vi "DEMO.vi"() -> ()   [LabVIEW 2013]
doc: "Use this template to build a producer/consumer design pattern with events to produce queue items. Use this design pattern instead of the User Interface Event Handler pattern for user interfaces when you want to execute code asynchronously in response to an event without slowing the user interface responsiveness."
uses:
  GumballMachine.lvclass/GumballMachine.lvclass
  ActionMark.ctl
panel:
  in  "Charge":bool
  out "ProcessMessage":string
  in  "TurnCrank":bool
  in  "EjectCoin":bool
  in  "InsertCoin":bool
  # "狀態模式簡例"
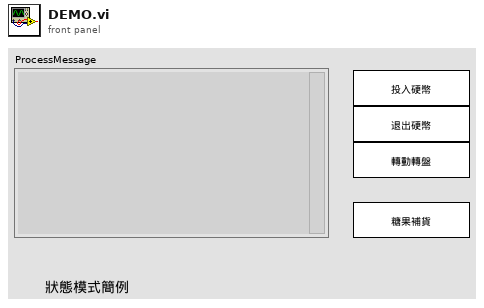
[diagram p1: front panel]
types:
  T1 = typedef "ActionMark.ctl" = enum16{"投入硬幣", "退回硬幣", "轉動轉盤", "糖果補貨"}
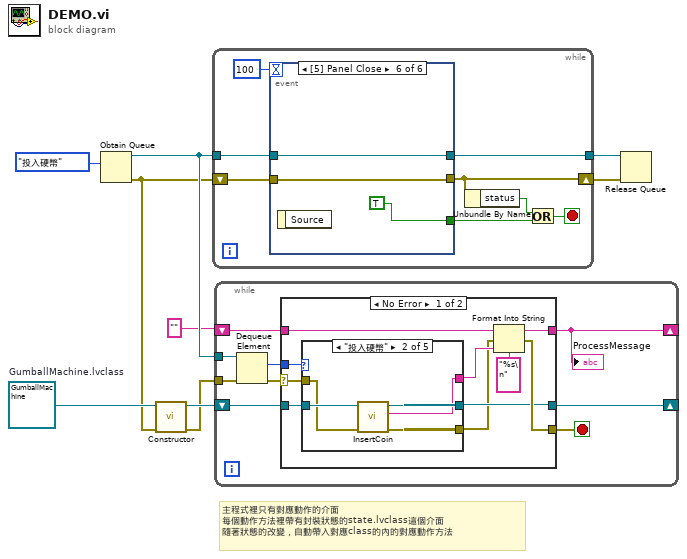
[diagram p0: block diagram]
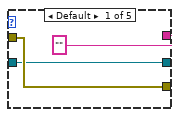
[diagram p2: hidden frame]
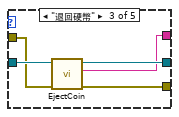
[diagram p3: hidden frame]
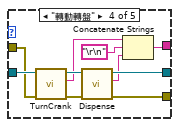
[diagram p4: hidden frame]
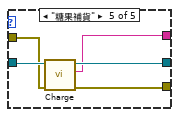
[diagram p5: hidden frame]
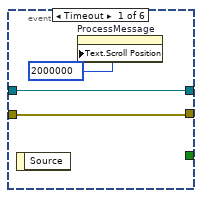
[diagram p7: hidden frame]
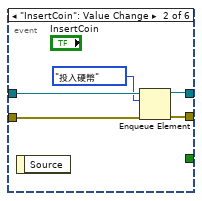
[diagram p8: hidden frame]
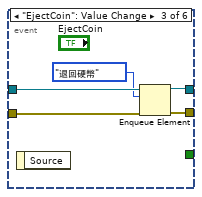
[diagram p9: hidden frame]
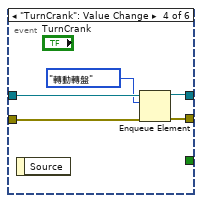
[diagram p10: hidden frame]
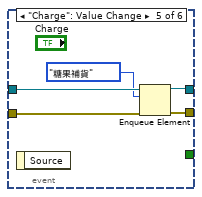
[diagram p11: hidden frame]
diagram:
  w5 = refnum<class "GumballMachine.lvclass"> refnum  # GumballMachine.lvclass
  # "主程式裡只有對應動作的介面\n每個動作方法裡帶有封裝狀態的state.lvclass這個介面\n隨著狀態的改變，自動帶入對應class的內的對應動作方法"
  n1 = Obtain Queue(element data type=ActionMark."投入硬幣" ("State")) -> (queue out=w8:refnum<queue>, error out=w2:errorcluster)  [unwired: 4 in, 1 out]
  n2 = call "Constructor.vi"("error in (no error)"=w2, "GumballMachine in"=w5) -> ("error out"=w3:errorcluster, "GumballMachine out"=w4:refnum<class "GumballMachine.lvclass">)  [unwired: 8 in]
  n3 = while {
    shift-right: [w13] -> w9
    shift-left: w2 -> [w16]
    tunnel: w8 -> [w17]
    tunnel: [w11] -> w6
    stop <- w14 stop-if-true
    n4 = event shown="[5] Panel Close" {
      selector: _ -> [_ _ _ _ _ _]
      dyn-events: _ -> [_ _ _ _ _ _]
      timeout: 100 -> [_ _ _ _ _ _]
      tunnel: w17 -> [w19 w25 w30 w35 w40 w41]
      tunnel: w16 -> [w20 w24 w29 w34 w39 w43]
      tunnel: [w20 w23 w28 w33 w38 w43] -> w13
      tunnel: [_ _ _ _ _ TRUE ("stop")] -> w15
      tunnel: [w19 w21 w26 w31 w36 w41] -> w11
      event Timeout {
        n5 = event-data() -> ()  [unwired: 1 in, 1 out]
        n6 = property on="ProcessMessage" class="Str"("Text.Scroll Position"=u32 2000000) -> ()  [unwired: 2 in, 2 out]
      }
      event "InsertCoin": Value Change {
        n7 = event-data() -> ()  [unwired: 1 in, 1 out]
        n8 = Enqueue Element(queue=w25, element=ActionMark."投入硬幣" ("State"), error in (no error)=w24) -> (queue out=w21:refnum<queue>, error out=w23:errorcluster)  [unwired: 1 in, 1 out]
      }
      event "EjectCoin": Value Change {
        n9 = event-data() -> ()  [unwired: 1 in, 1 out]
        n10 = Enqueue Element(queue=w30, element=ActionMark."退回硬幣" ("State"), error in (no error)=w29) -> (queue out=w26:refnum<queue>, error out=w28:errorcluster)  [unwired: 1 in, 1 out]
      }
      event "TurnCrank": Value Change {
        n11 = event-data() -> ()  [unwired: 1 in, 1 out]
        n12 = Enqueue Element(queue=w35, element=ActionMark."轉動轉盤" ("State"), error in (no error)=w34) -> (queue out=w31:refnum<queue>, error out=w33:errorcluster)  [unwired: 1 in, 1 out]
      }
      event "Charge": Value Change {
        n13 = event-data() -> ()  [unwired: 1 in, 1 out]
        n14 = Enqueue Element(queue=w40, element=ActionMark."糖果補貨" ("State"), error in (no error)=w39) -> (queue out=w36:refnum<queue>, error out=w38:errorcluster)  [unwired: 1 in, 1 out]
      }
      event Panel Close {
        n15 = event-data() -> ()  [unwired: 1 in, 1 out]
      }
    }
    n16 = Unbundle By Name(w13) -> ("status"=w12:bool)
    n17 = Or(x=w12, y=w15) -> (x .or. y?=w14:bool)
  }
  n18 = while {
    tunnel: w8 -> [w52]
    tunnel: w3 -> [w49]
    shift-right: [w47] -> _
    shift-left: w4 -> [w48]
    shift-right: [w44] -> _
    shift-left: "" -> [w45]
    stop <- w46 stop-if-true
    n19 = Dequeue Element(queue=w52, error in (no error)=w49) -> (element=w50:T1, error out=w51:errorcluster)  [unwired: 1 in, 2 out]
    n20 = case shown="No Error" w51 {
      selector: w51 -> [w60 w93]
      tunnel: w50 -> [w62 _]
      tunnel: w48 -> [w61 w92]
      tunnel: [w54 w92] -> w47
      tunnel: [w55 w93] -> w46
      tunnel: w45 -> [w57 w91]
      tunnel: [w59 w91] -> w44
      frame No Error {
        n21 = case shown="\"投入硬幣\"" w62 {
          tunnel: w61 -> [w64 w70 w75 w85 w90]
          tunnel: [w64 w69 w72 w83 w87] -> w54
          tunnel: w60 -> [w65 w68 w74 w84 w89]
          tunnel: [w65 w67 w73 w82 w88] -> w53
          tunnel: ["" w66 w71 w79 w86] -> w56
          frame Default {
          }
          frame "投入硬幣" {
            n22 = call-dynamic "InsertCoin.vi"("error in (no error)"=w68, "GumballMachine in"=w70) -> ("error out"=w67:errorcluster, "ProcessMessage"=w66:string, "GumballMachine out"=w69:refnum<class "GumballMachine.lvclass">)  [unwired: 7 in]
          }
          frame "退回硬幣" {
            n23 = call-dynamic "EjectCoin.vi"("error in (no error)"=w74, "GumballMachine in"=w75) -> ("error out"=w73:errorcluster, "ProcessMessage"=w71:string, "GumballMachine out"=w72:refnum<class "GumballMachine.lvclass">)  [unwired: 7 in]
          }
          frame "轉動轉盤" {
            n24 = call-dynamic "TurnCrank.vi"("error in (no error)"=w84, "GumballMachine in"=w85) -> ("error out"=w80:errorcluster, "ProcessMessage"=w78:string, "GumballMachine out"=w81:refnum<class "GumballMachine.lvclass">)  [unwired: 7 in]
            n25 = call-dynamic "Dispense.vi"("error in (no error)"=w80, "GumballMachine in"=w81) -> ("error out"=w82:errorcluster, "ProcessMessage"=w77:string, "GumballMachine out"=w83:refnum<class "GumballMachine.lvclass">)  [unwired: 7 in]
            n26 = Concatenate Strings(w78, "\r\n", w77) -> (w79:string)
          }
          frame "糖果補貨" {
            n27 = call-dynamic "Charge.vi"("error in (no error)"=w89, "GumballMachine in"=w90) -> ("error out"=w88:errorcluster, "ProcessMessage"=w86:string, "GumballMachine out"=w87:refnum<class "GumballMachine.lvclass">)  [unwired: 7 in]
          }
        }
        n28 = Format Into String(format string="%s\n", initial string=w57, error in=w53, w56) -> (resulting string=w59:string, error out=w55:errorcluster)
      }
      frame Error {
      }
    }
    "ProcessMessage" <- w44
  }
  n29 = Release Queue(queue=w6, error in (no error)=w9) -> ()  [unwired: 1 in, 3 out]
